vi "MachineStatus.vi"(4 "Keyboard 2":bool, 8 "Error":errorcluster, 11 "notifier in":refnum<notifier>) -> (0 "outError":errorcluster)   [LabVIEW 2017]
uses:
  GV/All Inputs.vi
  GV/MachineStatusGV.vi
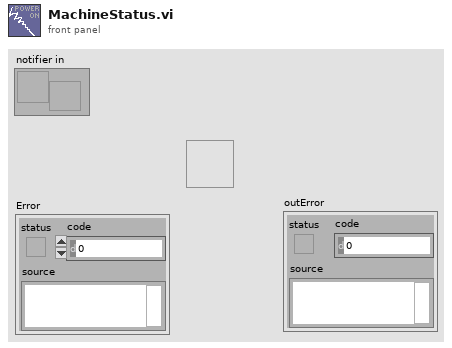
[diagram p1: front panel]
types:
  T1 = typedef "All Inputs.ctl" = cluster{"DI":cluster{"Machine ON":bool, "E-Stop":bool, "Pressure":bool, "Start":bool, "Safety Curtain":bool, "RS Load UP Rear":bool, "RS Load UP Front":bool, "RS Load DN Rear":bool, "RS Load DN Front":bool, "RS Loadcell Rear":bool, "RS Loadcell Front":bool, "Reject Sensor 1":bool, "Reject Sensor 2":bool, "Door SW Reject":bool}, "AI":cluster{"Force":dbl[], "Stroke":dbl[], "CurrentMon":dbl[]}, "SACB Inputs":T2}
  T2 = typedef "SACB DI.ctl" = cluster{"RS ClampTop Front":bool, "RS ClampBottom Front":bool, "RS ClampMotorLH Front":bool, "RS ClampMotorRH Front":bool, "IPS PartPresenceTop LH":bool, "IPS PartPresenceBottom LH":bool, "IPS PartPresenceTop RH":bool, "IPS PartPresenceBottom RH":bool, "IPS LoadEngaged 1":bool, "IPS LoadEngaged 2":bool, "C10":bool, "C11":bool, "C12":bool, "C13":bool, "C14":bool, "C15":bool}
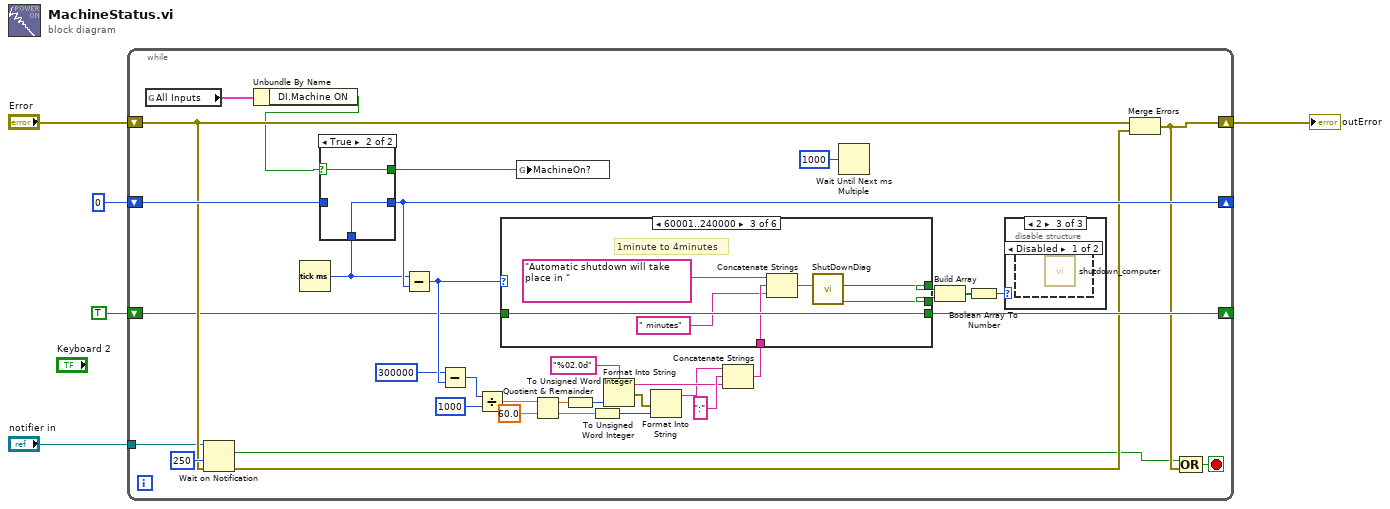
[diagram p0: block diagram]
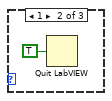
[diagram p3: hidden frame]
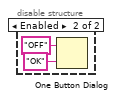
[diagram p4: hidden frame]
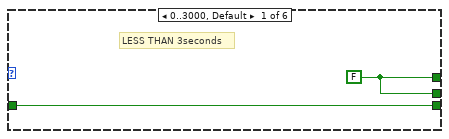
[diagram p5: hidden frame]
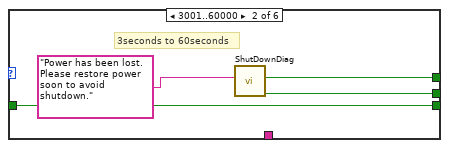
[diagram p6: hidden frame]
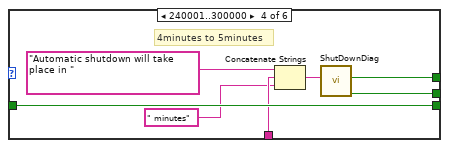
[diagram p7: hidden frame]
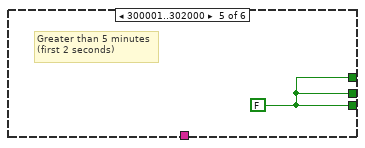
[diagram p8: hidden frame]
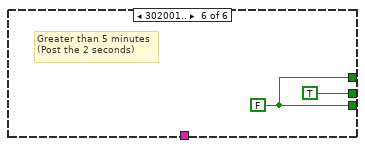
[diagram p9: hidden frame]
diagram:
  n1 = while {
    shift-right: [w39] -> _
    shift-left: TRUE ("Boolean") -> [w7]
    shift-right: [w40] -> _
    shift-left: u32 0 ("MillisecondValue") -> [w41]
    shift-right: [w11] -> w2
    shift-left: "Error" -> [w14]
    tunnel: "notifier in" -> [w9]
    stop <- w13 stop-if-true
    n2 = global read "All Inputs.vi" "All Inputs"() -> (w8:T1)
    n3 = Wait on Notification(notifier=w9, timeout in ms (-1)=250, error in (no error)=w14) -> (notification=w10:bool, error out=w12:errorcluster)  [unwired: 1 in, 2 out]
    n4 = Unbundle By Name(w8) -> ("DI.Machine ON"=w6:bool)
    n5 = Tick Count (ms)() -> (millisecond timer value=w37:u32)
    n6 = case shown="True" w6 {
      selector: w6 -> [w68 w70]
      tunnel: w41 -> [w69 _]
      tunnel: w37 -> [_ w71]
      tunnel: [w69 w71] -> w40
      tunnel: [w68 w70] -> w21
      frame False {
      }
      frame True {
      }
    }
    n7 = Subtract(x=w37, y=w40) -> (x-y=w25:u32)
    n8 = Subtract(x=u32 300000 ("y"), y=w25) -> (x-y=w26:u32)
    n9 = Divide(x=w26, y=u32 1000) -> (x/y=w35:dbl)
    n10 = global write "MachineStatusGV.vi" "MachineOn?"(w21) -> ()
    n11 = Quotient & Remainder(x=w35, y=60.0) -> (x-y*floor(x/y)=w31:dbl, floor(x/y)=w29:dbl)
    n12 = To Unsigned Word Integer(number=w31) -> (unsigned 16bit integer=w30:u16)
    n13 = To Unsigned Word Integer(number=w29) -> (unsigned 16bit integer=w28:u16)
    n14 = Format Into String(format string="%02.0d", w30) -> (resulting string=w23:string, error out=w33:errorcluster)  [unwired: 2 in]
    n15 = Format Into String(error in=w33, w28) -> (resulting string=w22:string)  [unwired: 2 in, 1 out]
    n16 = Concatenate Strings(w22, ":" ("string"), w23) -> (w27:string)
    n17 = case shown="60001..240000" w25 {
      tunnel: [w46 w50 w57 w64 w65 w67] -> w39
      tunnel: w7 -> [w46 w50 w57 w64 _ _]
      tunnel: w27 -> [_ _ w54 w61 _ _]
      tunnel: [w45 w48 w51 w59 w65 TRUE ("ShutDownNOW?")] -> w18
      tunnel: [w45 w49 w52 w58 w65 w67] -> w19
      frame 0..3000, Default {
        w45 = FALSE ("Exit?")
        # "LESS THAN 3seconds"
      }
      frame 3001..60000 {
        # "3seconds to 60seconds"
        n18 = call "ShutDownDiag.vi"("Caption.Text"="Power has been lost. Please restore power soon to avoid shutdown.") -> ("ShutDownNOW?"=w48:bool, "Exit?"=w49:bool)  [unwired: 9 in]
      }
      frame 60001..240000 {
        # "1minute to 4minutes"
        n19 = Concatenate Strings("Automatic shutdown will take place in " ("Caption.Text"), w54, " minutes" ("string")) -> (w55:string)
        n20 = call "ShutDownDiag.vi"("Caption.Text"=w55) -> ("ShutDownNOW?"=w51:bool, "Exit?"=w52:bool)  [unwired: 9 in]
      }
      frame 240001..300000 {
        # "4minutes to 5minutes"
        n21 = Concatenate Strings("Automatic shutdown will take place in " ("Caption.Text"), w61, " minutes" ("string")) -> (w62:string)
        n22 = call "ShutDownDiag.vi"("Caption.Text"=w62) -> ("ShutDownNOW?"=w59:bool, "Exit?"=w58:bool)  [unwired: 9 in]
      }
      frame 300001..302000 {
        w65 = FALSE
        # "Greater than 5 minutes\n(first 2 seconds)"
      }
      frame 302001.. {
        w67 = FALSE
        # "Greater than 5 minutes\n(Post the 2 seconds)"
      }
    }
    n23 = Wait Until Next ms Multiple(millisecond multiple=u32 1000) -> ()  [unwired: 1 out]
    n24 = Build Array(w19, w18) -> (w17:bool[])
    n25 = Boolean Array To Number(Boolean array=w17) -> (number=w16:u32)
    n26 = case shown="2" w16 {
      frame 0, Default {
      }
      frame 1 {
        n27 = Quit LabVIEW(quit? (T)=TRUE) -> ()
      }
      frame 2 {
        n28 = disable-structure shown="Disabled" {
          frame Disabled {
            n29 = call "shutdown_computer.vi"() -> ()  [unwired: 1 in]
          }
          frame Enabled {
            n30 = One Button Dialog(message="OFF", button name ("OK")="OK") -> ()  [unwired: 1 out]
          }
        }
      }
    }
    n31 = Merge Errors(w14, w12) -> (w11:errorcluster)
    n32 = Compound Arithmetic op=OR(w10, w11) -> (w13:bool)
  }
  "outError" <- w2
